vi "rs3 Advanced set color correction3.vi"(8 "error in (no error)":errorcluster, 10 "STColorCorrection input":T1={"colorCorrection 1"=0.15039062, "colorCorrection 2"=0.46484375, "colorCorrection 3"=0.46484375, "colorCorrection 4"=3.9189453, "colorCorrection 5"=3.8027344, "colorCorrection 6"=3.5986328, "colorCorrection 7"=3.5986328, "colorCorrection 8"=0.99902344, "colorCorrection 9"=1.2910156, "colorCorrection 10"=3.381836, "colorCorrection 11"=3.381836, "colorCorrection 12"=3.944336}, 11 "device in":u64) -> (0 "error out":errorcluster, 1 "error":u64, 3 "Dev out":u64)   [LabVIEW 2023]
doc: "This sets the color correction matrix. It does NOT affect the depth calculations."
panel:
  # "RS3 Adv. Set Color Correct."
  # "(C) 2017 Intel Corp.,  AGJ"
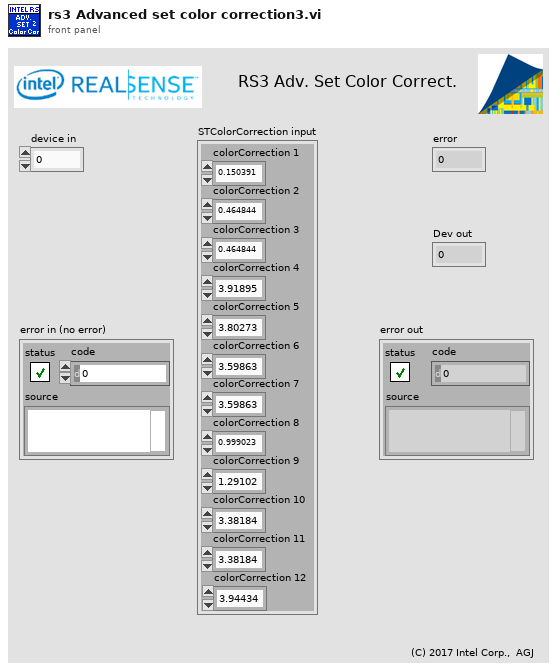
[diagram p1: front panel]
types:
  T1 = cluster{"colorCorrection 1":sgl, "colorCorrection 2":sgl, "colorCorrection 3":sgl, "colorCorrection 4":sgl, "colorCorrection 5":sgl, "colorCorrection 6":sgl, "colorCorrection 7":sgl, "colorCorrection 8":sgl, "colorCorrection 9":sgl, "colorCorrection 10":sgl, "colorCorrection 11":sgl, "colorCorrection 12":sgl}
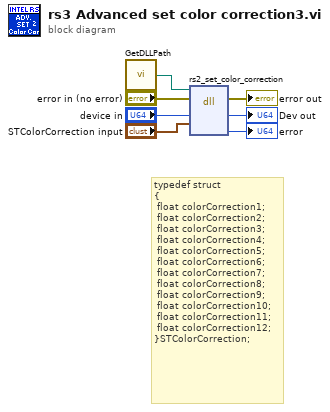
[diagram p0: block diagram]
diagram:
  # "typedef struct\n{\n\tfloat colorCorrection1;\n\tfloat colorCorrection2;\n\tfloat colorCorrection3;\n\tfloat colorCorrection4;\n\tfloat colorCorrection5;\n\tfloat colorCorrection6;\n\tfloat colorCorrection7;\n\tfloat colorCorrection8;\n\tfloat colorCorrection9;\n\tfloat colorCorrection10;\n\tfloat colorCorrection11;\n\tfloat colorCorrection12;\n}STColorCorrection;"
  n1 = call "GetDLLPath.vi"() -> ("DLL Path"=w1:path)
  n2 = dll-call lib="C:/STEAMSyndicate/RealSenseWrappers/VI Wrappers (add ons) Public/RealSense/realsense2.dll" fn="rs2_set_color_correction"(path in=w1, error in="error in (no error)", "device"="device in", "color correction"="STColorCorrection input") -> (error out=→"error out":errorcluster, "device"=→"Dev out":u64, "error"=→"error":u64)  [unwired: 4 in, 1 out]
